vi "fds1 (SubVI).vi"(11 "Compressor\nTemp.":dbl) -> (0 "cpair":dbl, 3 "gammair":dbl)   [LabVIEW 2019]
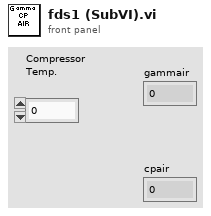
[diagram p1: front panel]
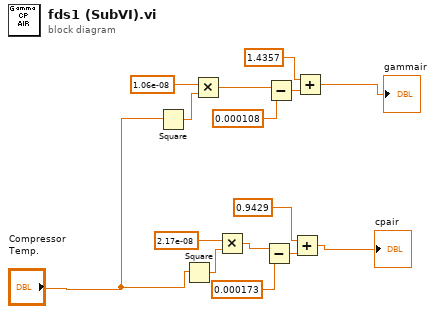
[diagram p0: block diagram]
diagram:
  n1 = Square(x="Compressor\nTemp.") -> (x^2=w11:dbl)
  n2 = Square(x="Compressor\nTemp.") -> (x^2=w6:dbl)
  n3 = Multiply(x=1.06e-08, y=w11) -> (x*y=w12:dbl)
  n4 = Multiply(x=2.17e-08, y=w6) -> (x*y=w5:dbl)
  n5 = Subtract(x=w5, y=0.000173) -> (x-y=w3:dbl)
  n6 = Subtract(x=w12, y=0.000108) -> (x-y=w14:dbl)
  n7 = Add(x=0.9429, y=w3) -> (x+y=→"cpair":dbl)
  n8 = Add(x=1.4357, y=w14) -> (x+y=→"gammair":dbl)
